vi "Emballage_BDD_GVF_Reference.vi"(0 "SetGet":T1=enum."get", 5 "ref Piece IN":refnum<vi>, 11 "Error in":errorcluster caption="Error in (no error)") -> (6 "ref piece OUT":refnum<vi>, 15 "Error out":errorcluster)   [LabVIEW 2020]
uses:
  Modules/FS/60_FS_Controles/60_FS_SetGet.ctl
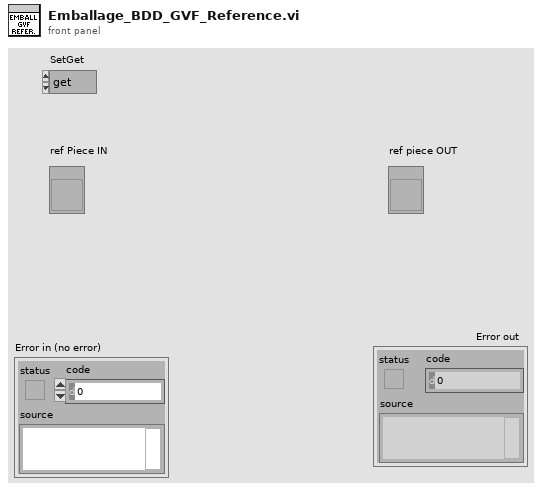
[diagram p1: front panel]
types:
  T1 = typedef "60_FS_SetGet.ctl" = enum16{"set", "get"}
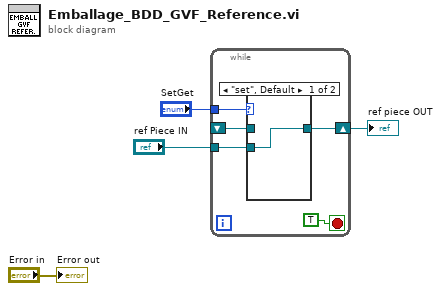
[diagram p0: block diagram]
diagram:
  n1 = while {
    tunnel: "SetGet" -> [w8]
    tunnel: "ref Piece IN" -> [w6]
    shift-right: [w7] -> w2
    shift-left: _ -> [w5]
    stop <- TRUE stop-if-true
    n2 = case shown="\"set\", Default" w8 {
      tunnel: [w10 w11] -> w7
      tunnel: w6 -> [w10 _]
      tunnel: w5 -> [_ w11]
      frame "set", Default {
      }
      frame "get" {
      }
    }
  }
  "ref piece OUT" <- w2
  "Error out" <- "Error in"
